vi "Send Configure Runt Trigger Source [RT].vi"(6 "runt high threshold (4.0 V)":dbl[unit]=4.0 format="%.3f", 7 "Message Priority (Normal)":T1=enum."Normal", 8 "error in (no error)":errorcluster, 9 "runt low threshold (1.0 V)":dbl[unit]=1.0 format="%.3f", 10 "trigger source (\"CHANNEL1\")":string(combo)="CHANNEL1", 11 "Message Enqueuer":refnum<class "Message Enqueuer.lvclass">) -> (0 "error out":errorcluster, 3 "Message Enqueuer out":refnum<class "Message Enqueuer.lvclass">)   [LabVIEW 2015, in "CS++Scope.lvlib" / "Configure Runt Trigger Source [RT] Msg.lvclass"]
doc: "Sends the <B>CS++Scope.lvlib:Configure Runt Trigger Source [RT] Msg.lvclass</B> message.\n\n<B>CS++Scope.lvlib:CS++Scope.lvclass:Configure Runt Trigger Source [RT].vi</B> Description:\n\nThis VI configures the runt trigger. A runt trigger occurs when the trigger signal you specify with the Runt Trigger Source parameter crosses one of the runt thresholds twice without crossing the other runt threshold. You specify the runt thresholds with the Runt Low Threshold and Runt High Threshold parameters. You specify the polarity of the runt with the Runt Polarity parameter.\n\nNote \n(1) This VI affects instrument behavior only if the trigger type is\n IVISCOPE_VAL_RUNT_TRIGGER. Call the IviScope Configure Trigger\n and IviScope Configure Trigger Coupling VIs to set the trigger type and\n trigger coupling before calling this VI.\n\n(2) This VI is part of the IviScopeRuntTrigger [RT] extension group."
uses:
  Configure Runt Trigger Source [RT] Msg.lvclass
  <vilib>/ActorFramework/Message Enqueuer/Message Enqueuer.lvclass
  <vilib>/ActorFramework/Message Enqueuer/Message Priority.ctl
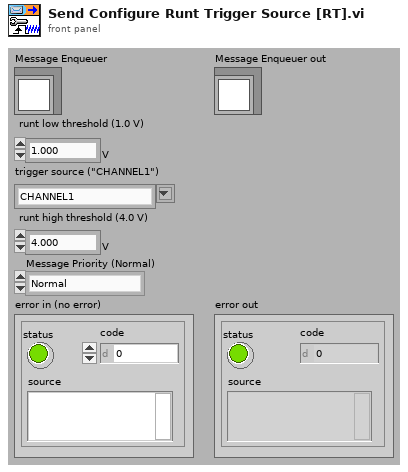
[diagram p1: front panel]
types:
  T1 = typedef "Actor Framework.lvlib/Message Enqueuer.lvclass/Message Priority.ctl" = enum16{"Low", "Normal", "High"}
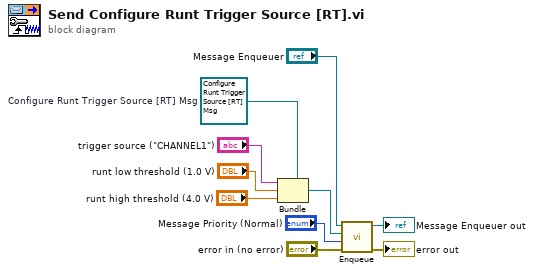
[diagram p0: block diagram]
diagram:
  w4 = refnum<class "Configure Runt Trigger Source [RT] Msg.lvclass"> refnum  # Configure Runt Trigger Source [RT] Msg
  n1 = Bundle(cluster=w4, "trigger source (\"CHANNEL1\")", "runt low threshold (1.0 V)", "runt high threshold (4.0 V)") -> (w7:refnum<class "Configure Runt Trigger Source [RT] Msg.lvclass">)
  n2 = call <vilib>:"Enqueue.vi"("error in (no error)"="error in (no error)", "Message Priority (Normal)"="Message Priority (Normal)", "Message"=w7, "Message Enqueuer in"="Message Enqueuer") -> ("error out"=→"error out":errorcluster, "Message Enqueuer out"=→"Message Enqueuer out":refnum<class "Message Enqueuer.lvclass">)  [unwired: 6 in]
